vi "Kalman Calculation.vi"(6 "R":T1=[[0.1, 0.0, 0.0], [0.0, 0.1, 0.0], [0.0, 0.0, 0.1]], 7 "Use Observation":bool=TRUE, 8 "intervalo":dbl=1.0, 9 "Pk-1|k-1":T1, 10 "x_k-1|k-1":T1=[[0.0, 0.0, 0.0], [0.0, 0.0, 0.0], [0.0, 0.0, 0.0]], 11 "z_k":T1) -> (1 "Conf":dbl, 2 "Pk|k":T1, 3 "x_k|k":T1)   [LabVIEW 2017]
uses:
  <vilib>/Analysis/Matrix/NI_Matrix.lvlib
  <vilib>/Analysis/NI_AALBase.lvlib
  <vilib>/Analysis/Matrix/Numeric/Multiply/Multiply - RM,RM.vi
  <vilib>/Analysis/Matrix/Numeric/Add/Add - RM,RM.vi
  <vilib>/Analysis/baseanly.llb/Real Inverse Matrix.vi
  <vilib>/Analysis/Matrix/Datatypes/RealMatrix.ctl
  <vilib>/Analysis/Matrix/Numeric/Subtract/Subtract - RM,RM.vi
  <vilib>/Analysis/NI_AALPro.lvlib
  <vilib>/Analysis/_algsub.llb/Real Matrix Norm.vi
panel:
  out "K_k":T1
  out "Inverse Matrix":T1
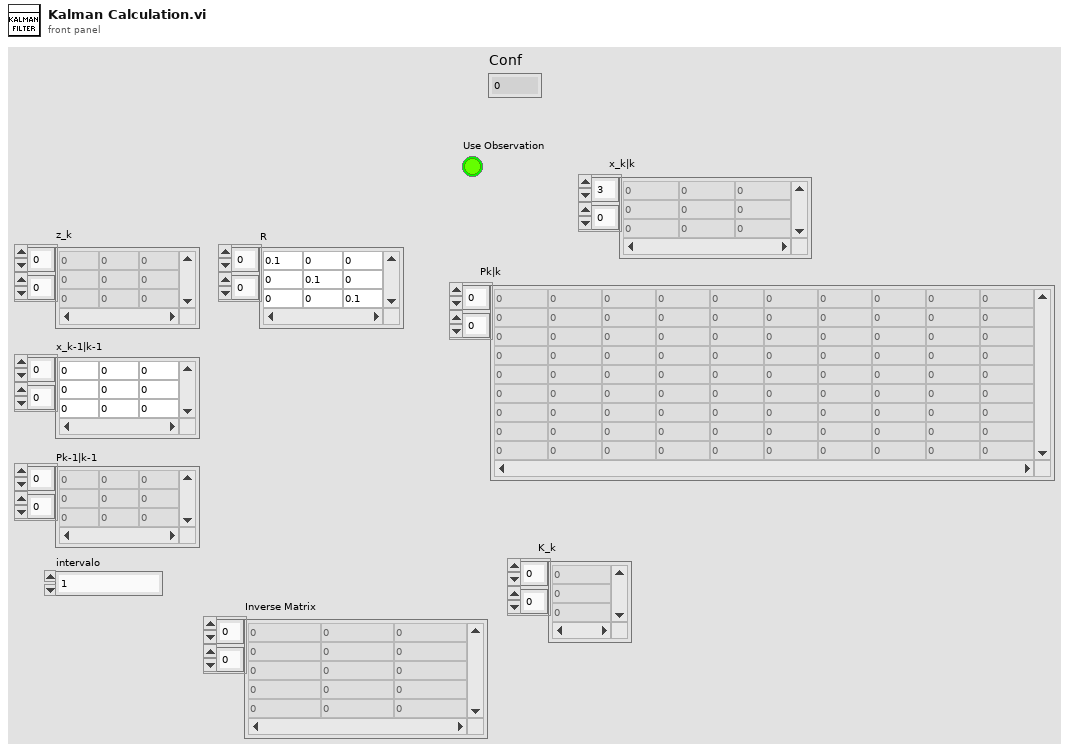
[diagram p1: front panel]
types:
  T1 = typedef "NI_Matrix.lvlib/RealMatrix.ctl" = dbl[][]
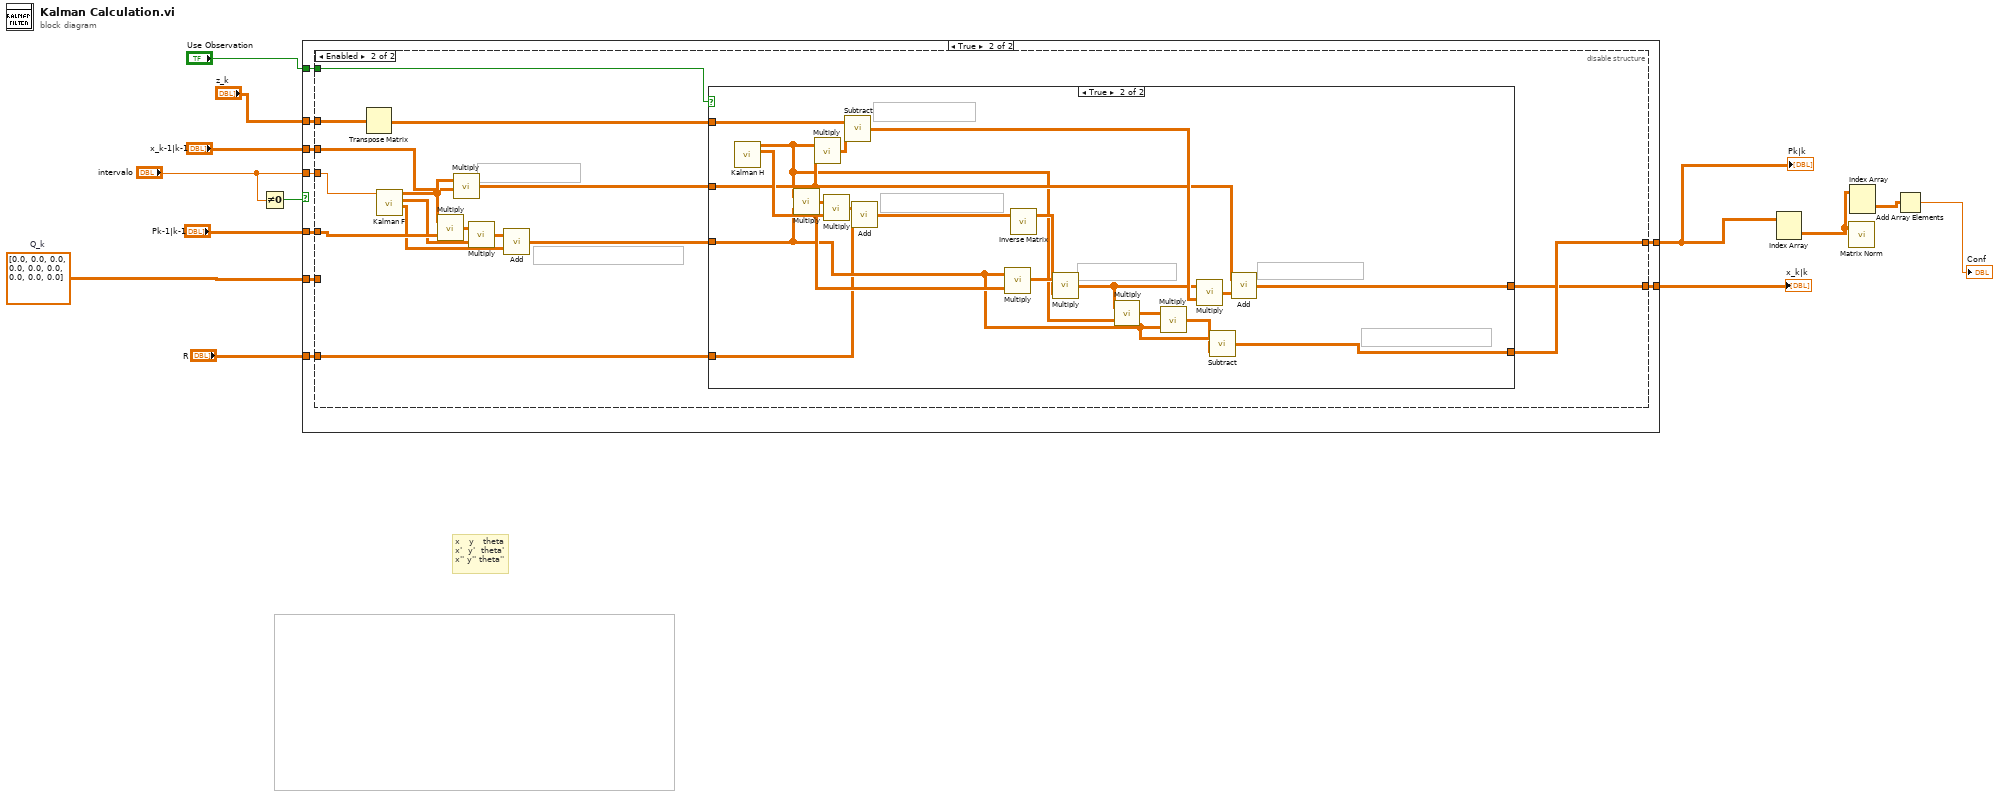
[diagram p0: block diagram]
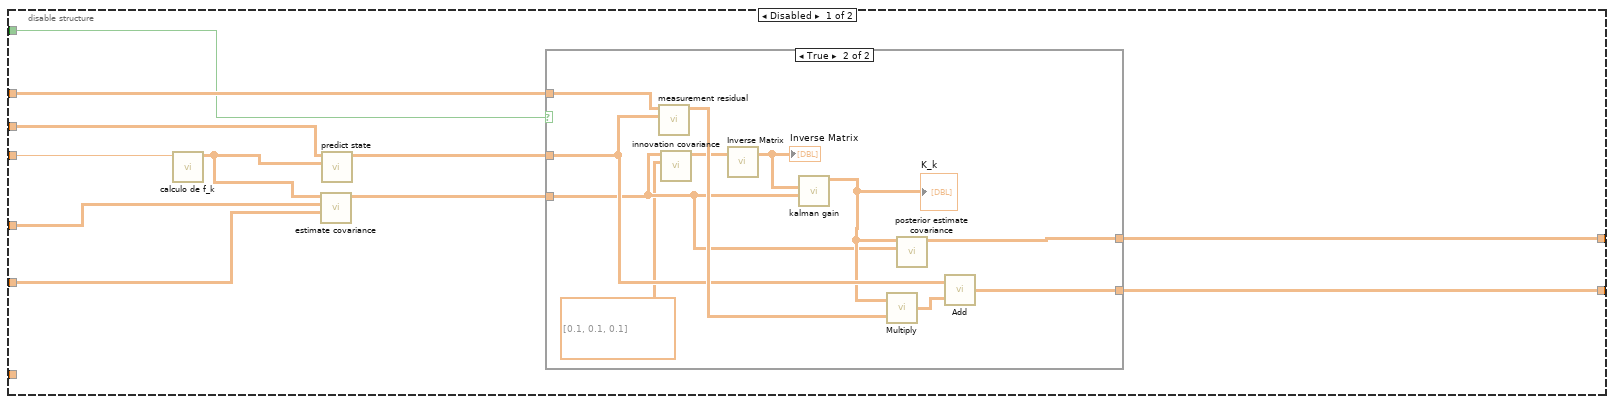
[diagram p3: hidden frame]
diagram:
  w9 = T1 [[0.0, 0.0, 0.0], [0.0, 0.0, 0.0], [0.0, 0.0, 0.0]]  # Q_k
  # "x   y   theta\nx'  y'  theta'\nx'' y'' theta''"
  n1 = Not Equal To 0?(x="intervalo") -> (x != 0?=w10:bool)
  n2 = case shown="True" w10 {
    tunnel: "intervalo" -> [_ w24]
    tunnel: [w15 w23] -> w1
    tunnel: "Pk-1|k-1" -> [w14 w22]
    tunnel: "x_k-1|k-1" -> [w15 w20]
    tunnel: [w14 w21] -> w11
    tunnel: w9 -> [_ w19]
    tunnel: "z_k" -> [_ w18]
    tunnel: "Use Observation" -> [_ w17]
    tunnel: "R" -> [_ w16]
    frame False {
    }
    frame True {
      n3 = disable-structure shown="Enabled" {
        disable-tunnel: w24 -> [w35 w64]
        disable-tunnel: [w32 w53] -> w23
        disable-tunnel: w22 -> [w31 w63]
        disable-tunnel: [w30 w54] -> w21
        disable-tunnel: w20 -> [w29 w51]
        disable-tunnel: w19 -> [w27 _]
        disable-tunnel: w18 -> [w26 w58]
        disable-tunnel: w17 -> [w25 w49]
        disable-tunnel: w16 -> [_ w50]
        frame Disabled {
          n4 = call "calculo de f_k.vi"("iteração"=w35) -> ("F_k"=w28:T1)  [unwired: 10 in]
          n5 = call "estimate covariance.vi"("Q_k"=w27, "Pk-1|k-1"=w31, "F_k"=w28) -> ("Pk|k-1"=w33:T1)  [unwired: 8 in]
          n6 = call "predict state.vi"("F_k"=w28, "x_k-1|k-1"=w29) -> ("x_k|k-1"=w34:T1)  [unwired: 9 in]
          n7 = case shown="True" w25 {
            tunnel: [w37 w47] -> w32
            tunnel: w34 -> [w37 w45]
            tunnel: [w36 w42] -> w30
            tunnel: w33 -> [w36 w40]
            tunnel: w26 -> [_ w39]
            frame False {
            }
            frame True {
              n8 = call "measurement residual.vi"("x_k|k-1"=w45, "z_k"=w39) -> ("y~_k"=w46:T1)  [unwired: 9 in]
              n9 = call "innovation covariance.vi"("R"=T1 [[0.1, 0.1, 0.1]], "Pk|k-1"=w40) -> ("S_k"=w44:T1)  [unwired: 8 in, 1 out]
              n10 = call-poly <vilib>:"Inverse Matrix.vi"("Input Matrix"=w44) -> ("Inverse Matrix"=w43:T1)  [unwired: 1 in, 1 out]
              "Inverse Matrix" <- w43
              n11 = call "kalman gain.vi"("Pk|k-1"=w40, "S^-1"=w43) -> ("K_k"=w41:T1)  [unwired: 9 in]
              "K_k" <- w41
              n12 = call-poly <vilib>:"Multiply.vi"("Real Matrix B"=w46, "Real Matrix A"=w41) -> ("A * B"=w48:T1)
              n13 = call "posterior estimate covariance.vi"("Pk|k-1"=w40, "K_k"=w41) -> ("Pk|k"=w42:T1)  [unwired: 9 in]
              n14 = call-poly <vilib>:"Add.vi"("Real Matrix B"=w48, "Real Matrix A"=w45) -> ("A + B"=w47:T1)
            }
          }
        }
        frame Enabled {
          n15 = Transpose Matrix(1:w58) -> (0:w57:T1)
          n16 = call "Kalman F.vi"("intervalo"=w64) -> ("Q"=w59:T1, "F'"=w61:T1, "F"=w52:T1)  [unwired: 8 in]
          n17 = call-poly <vilib>:"Multiply.vi"("Real Matrix B"=w63, "Real Matrix A"=w52) -> ("A * B"=w62:T1)
          n18 = call-poly <vilib>:"Multiply.vi"("Real Matrix B"=w51, "Real Matrix A"=w52) -> ("A * B"=w56:T1)
          n19 = call-poly <vilib>:"Multiply.vi"("Real Matrix B"=w61, "Real Matrix A"=w62) -> ("A * B"=w60:T1)
          n20 = call-poly <vilib>:"Add.vi"("Real Matrix B"=w59, "Real Matrix A"=w60) -> ("A + B"=w55:T1)
          n21 = case shown="True" w49 {
            tunnel: w57 -> [_ w85]
            tunnel: w56 -> [w66 w75]
            tunnel: w55 -> [w65 w71]
            tunnel: [w65 w69] -> w54
            tunnel: [w66 w68] -> w53
            tunnel: w50 -> [_ w67]
            frame False {
            }
            frame True {
              n22 = call "Kalman H.vi"() -> ("H'"=w80:T1, "H"=w73:T1)  [unwired: 10 in]
              n23 = call-poly <vilib>:"Multiply.vi"("Real Matrix B"=w71, "Real Matrix A"=w73) -> ("A * B"=w83:T1)
              n24 = call-poly <vilib>:"Multiply.vi"("Real Matrix B"=w75, "Real Matrix A"=w73) -> ("A * B"=w84:T1)
              n25 = call-poly <vilib>:"Multiply.vi"("Real Matrix B"=w80, "Real Matrix A"=w83) -> ("A * B"=w82:T1)
              n26 = call-poly <vilib>:"Subtract.vi"("Real Matrix B"=w84, "Real Matrix A"=w85) -> ("A - B"=w77:T1)
              n27 = call-poly <vilib>:"Add.vi"("Real Matrix B"=w67, "Real Matrix A"=w82) -> ("A + B"=w81:T1)
              n28 = call-poly <vilib>:"Multiply.vi"("Real Matrix B"=w80, "Real Matrix A"=w71) -> ("A * B"=w79:T1)
              n29 = call-poly <vilib>:"Inverse Matrix.vi"("Input Matrix"=w81) -> ("Inverse Matrix"=w78:T1)  [unwired: 1 in, 1 out]
              n30 = call-poly <vilib>:"Multiply.vi"("Real Matrix B"=w78, "Real Matrix A"=w79) -> ("A * B"=w74:T1)
              n31 = call-poly <vilib>:"Multiply.vi"("Real Matrix B"=w73, "Real Matrix A"=w74) -> ("A * B"=w72:T1)
              n32 = call-poly <vilib>:"Multiply.vi"("Real Matrix B"=w71, "Real Matrix A"=w72) -> ("A * B"=w70:T1)
              n33 = call-poly <vilib>:"Multiply.vi"("Real Matrix B"=w77, "Real Matrix A"=w74) -> ("A * B"=w76:T1)
              n34 = call-poly <vilib>:"Subtract.vi"("Real Matrix B"=w70, "Real Matrix A"=w71) -> ("A - B"=w69:T1)
              n35 = call-poly <vilib>:"Add.vi"("Real Matrix B"=w76, "Real Matrix A"=w75) -> ("A + B"=w68:T1)
            }
          }
        }
      }
    }
  }
  "Pk|k" <- w11
  "x_k|k" <- w1
  n36 = Index Array(array=w11) -> (element=w4:T1)  [unwired: 2 in]
  n37 = call-poly <vilib>:"Matrix Norm.vi"("Input Matrix"=w4) -> ()  [unwired: 1 in, 2 out]
  n38 = Index Array(array=w4) -> (element=w3:T1)  [unwired: 2 in]
  n39 = Add Array Elements(numeric array=w3) -> (sum=→"Conf":dbl)
